vi "FTW-JSON-Object-DeleteElement.vi"(0 "JSON Object":refnum<data-value>, 5 "Key":string, 11 "error in":errorcluster) -> (4 "JSON Object out":refnum<data-value>, 6 "Found and Removed?":bool, 15 "error out":errorcluster)   [LabVIEW 2015]
uses:
  core/FTW-JSON-Core-Structure.ctl
panel:
  # "Inputs"
  # "Outputs"
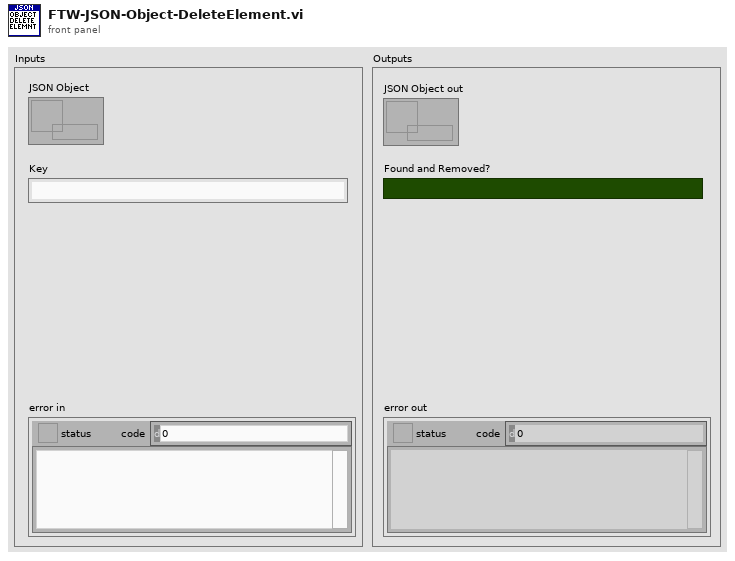
[diagram p1: front panel]
types:
  T1 = typedef "FTW-JSON-Core-Structure.ctl" = cluster{"JSON Object":i64, "Encoding Flags":i64, "Decoding Flags":i64}
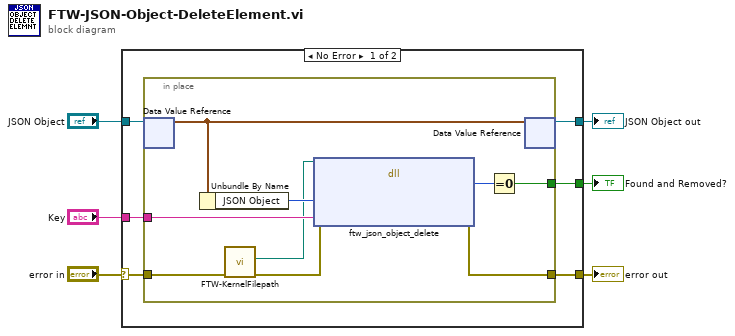
[diagram p0: block diagram]
diagram:
  n1 = case shown="No Error" "error in" {
    selector: "error in" -> [w12 w23]
    tunnel: [w10 w23] -> w6
    tunnel: [w7 w22] -> w4
    tunnel: "JSON Object" -> [w8 w22]
    tunnel: "Key" -> [w11 _]
    tunnel: [w9 _] -> w1
    frame No Error {
      n2 = in-place {
        in-place-border: w12 -> [w15]
        in-place-border: w11 -> [w21]
        in-place-border: [w20] -> w10
        in-place-border: [w18] -> w9
        n3 = in-place-dvr #1(w8) -> (w17:T1)  [unwired: 1 out]
        n4 = Unbundle By Name(w17) -> ("JSON Object"=w16:i64)
        n5 = call "FTW-KernelFilepath.vi"("error in"=w15) -> ("error out"=w14:errorcluster, "Library Filepath"=w13:path)  [unwired: 8 in, 1 out]
        n6 = dll-call lib="?" fn="ftw_json_object_delete"(path in=w13, error in=w14, "JSON Object Pointer"=w16, "Element Key"=w21) -> (error out=w20:errorcluster, "JSON Element Pointer"=w19:i64)  [unwired: 3 in, 1 out]
        n7 = Equal To 0?(x=w19) -> (x = 0?=w18:bool)
        n8 = in-place-dvr #1(w17) -> (w7:refnum<data-value>)  [unwired: 1 out]
      }
    }
    frame Error {
    }
  }
  "error out" <- w6
  "JSON Object out" <- w4
  "Found and Removed?" <- w1
